vi "MessageBase.setMessageTypeAndLength.vi"(8 "error in (no error)":errorcluster, 9 "MessageType":u8=33 format="%.0x", 10 "Length":u8=34, 11 "MessageBase in":refnum<class "MessageBase.lvclass">) -> (0 "error out":errorcluster, 3 "MessageBase out":refnum<class "MessageBase.lvclass">)   [LabVIEW 2022 SP3, in "MessageBase.lvclass"]
uses:
  MessageBase.lvclass
  FieldValue.ctl
  MessageBase.lvclass/MessageBase.ctl
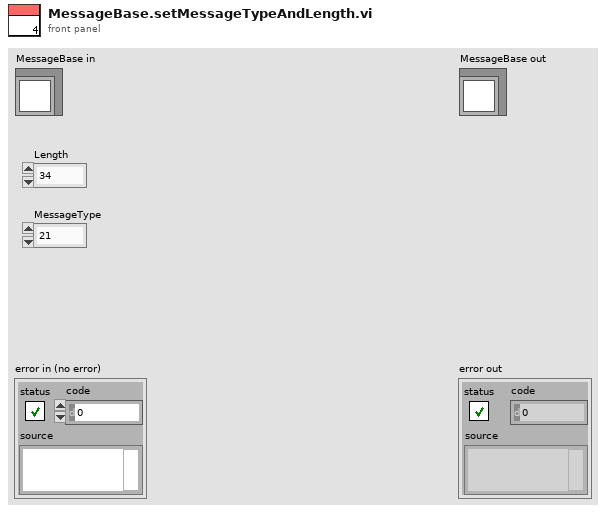
[diagram p1: front panel]
types:
  T1 = typedef "FieldValue.ctl" = variant
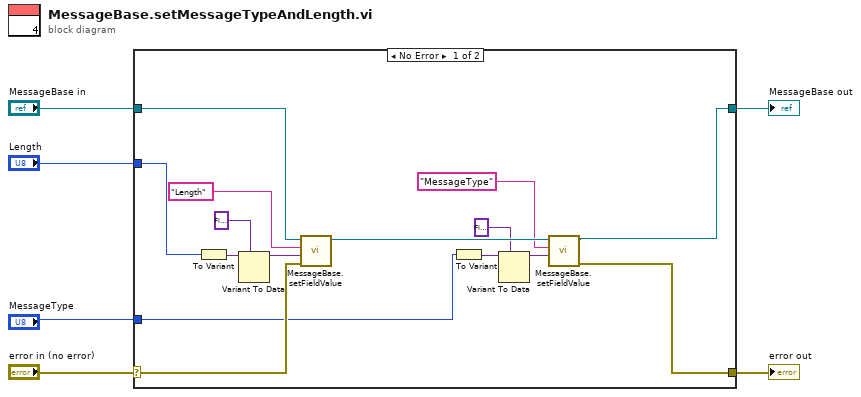
[diagram p0: block diagram]
diagram:
  n1 = case shown="No Error" "error in (no error)" {
    selector: "error in (no error)" -> [w12 w23]
    tunnel: [w11 w23] -> w5
    tunnel: [w7 w22] -> w3
    tunnel: "MessageBase in" -> [w9 w22]
    tunnel: "Length" -> [w10 _]
    tunnel: "MessageType" -> [w8 _]
    frame No Error {
      n2 = To Variant(anything=w10) -> (Variant=w17:variant)
      n3 = Variant To Data(type=T1 variant ("FieldValue"), Variant=w17) -> (data=w18:T1)  [unwired: 1 in, 1 out]
      n4 = call-dynamic "MessageBase.setFieldValue.vi"("error in (no error)"=w12, "Value"=w18, "FIeld.Name"="Length", "MessageBase in"=w9) -> ("MessageBase out"=w19:refnum<class "MessageBase.lvclass">)  [unwired: 6 in, 1 out]
      n5 = To Variant(anything=w8) -> (Variant=w20:variant)
      n6 = Variant To Data(type=T1 variant ("FieldValue"), Variant=w20) -> (data=w21:T1)  [unwired: 1 in, 1 out]
      n7 = call-dynamic "MessageBase.setFieldValue.vi"("Value"=w21, "FIeld.Name"="MessageType", "MessageBase in"=w19) -> ("error out"=w11:errorcluster, "MessageBase out"=w7:refnum<class "MessageBase.lvclass">)  [unwired: 7 in]
    }
    frame Error {
    }
  }
  "error out" <- w5
  "MessageBase out" <- w3
